vi "Subsistem Pengenalan Pola.vi"() -> ()   [LabVIEW 2011]
uses:
  <vilib>/vision/NI_Vision_Development_Module.lvlib
panel:
  in  "stop":bool
  in  "Color Plane":i32(ring)=1 items=["Red", "Green", "Blue", "Hue", "Saturation", "Luminance", "Value", "Intensity"]
  out "Objects":T1(array[cluster]) {"Aspect Ratio" format="%.2f"; "Orientation" format="%.2f"; "Area" format="%.2f"; "Object Center"."Y" format="%.2f"; "Object Center"."X" format="%.2f"}
  in  "Replace Value":sgl=255.0 format="%.2f"
  in  "Range":cluster{"Lower value":sgl, "Upper value":sgl}={"Lower value"=128.0, "Upper value"=255.0} {"Upper value" format="%.2f"; "Lower value" format="%.2f"}
  out "error vision 2":errorcluster
  in  "BERKAS / KAMERA":bool
  in  "Alamat Berkas":path=path "E:/D4 - TUGAS AKHIR/Programs/Praktikum/polman.png"
  out "Number of Objects":i32
  in  "Settings":T2={"Objects"=1, "Threshold"=128, "Reject Border"=FALSE, "Fill Holes"=FALSE, "Min Object Size"=FALSE, "Min Size"=100, "Max Object Size"=FALSE, "Max Size"=10000, "Show Search Area"=FALSE, "Show Center"=TRUE, "Show Bounding Box"=TRUE} {"Objects" items=["Bright Objects", "Dark Objects"]; "Threshold" min=1 max=999999999 step=1; "Max Size" min=1 max=999999999 step=1; "Min Size" min=1 max=999999999 step=1}
  out "Hasil \nKlasifikasi":T3(plugin-control)
  out "Hasil\nSegmentasi":T3(plugin-control)
  out "Citra \nHitam/Putih":T3(plugin-control)
  out "Citra Asli":T3(plugin-control)
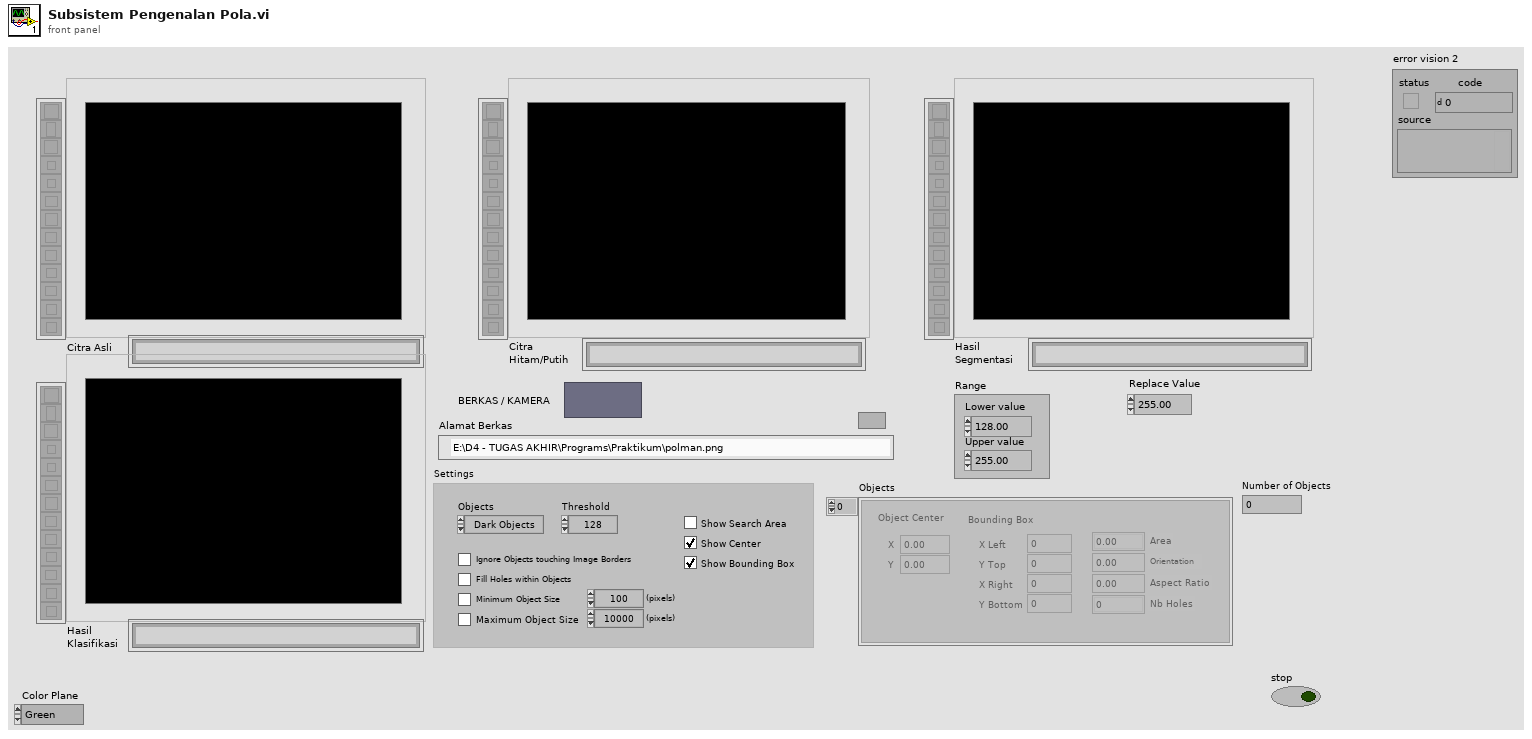
[diagram p1: front panel]
types:
  T1 = cluster{"Object Center":cluster{"X":sgl, "Y":sgl}, "Bounding Box":cluster{"X Left":i32, "Y Top":i32, "X Right":i32, "Y Bottom":i32}, "Area":sgl, "Orientation":sgl, "Aspect Ratio":sgl, "Nb Holes":i32}[]
  T2 = cluster{"Objects":u16, "Threshold":i32, "Reject Border":bool, "Fill Holes":bool, "Min Object Size":bool, "Min Size":i32, "Max Object Size":bool, "Max Size":i32, "Show Search Area":bool, "Show Center":bool, "Show Bounding Box":bool}
  T3 = typedef "IMAQ Image.ctl" = refnum<image>
  T4 = typedef "Image Type" = u32
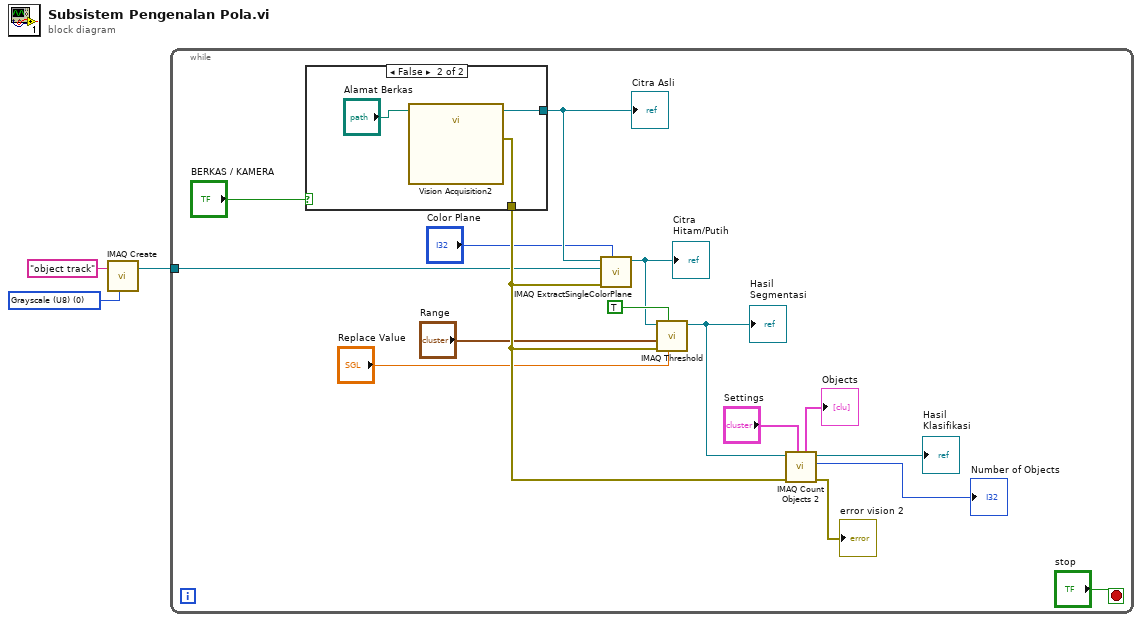
[diagram p0: block diagram]
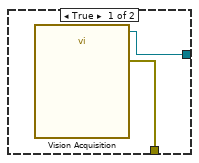
[diagram p2: hidden frame]
diagram:
  w2 = T4 0 items=["Grayscale (U8)", "Grayscale (I16)", "Grayscale (SGL)", "Complex (CSG)", "RGB (U32)", "HSL (U32)", "RGB (U64)", "Grayscale (U16)"] ("Image Type")
  n1 = call "IMAQ Create"("Image Name"="object track", "Image Type"=w2) -> ("New Image"=w1:T3)  [unwired: 3 in, 1 out]
  n2 = while {
    tunnel: w1 -> [w4]
    stop <- "stop" stop-if-true
    n3 = case shown="False" "BERKAS / KAMERA" {
      tunnel: [w20 w23] -> w19
      tunnel: [w21 w22] -> w13
      frame True {
        n4 = call "Vision Acquisition"() -> ("Image Out"=w20:T3, "error out"=w21:errorcluster)  [unwired: 25 in, 1 out]
      }
      frame False {
        n5 = call "Vision Acquisition2"("Image Path"="Alamat Berkas") -> ("Image Out"=w23:T3, "error out"=w22:errorcluster)  [unwired: 24 in, 1 out]
      }
    }
    "Citra Asli" <- w19
    n6 = call "IMAQ ExtractSingleColorPlane"("Color Plane"="Color Plane", "error in (no error)"=w13, "Image Dst"=w4, "Image Src"=w19) -> ("Image Dst Out"=w7:T3)  [unwired: 6 in, 1 out]
    "Citra \nHitam/Putih" <- w7
    n7 = call "IMAQ Threshold"("Replace Value"="Replace Value", "Keep/Replace Value (Replace)"=TRUE, "error in (no error)"=w13, "Range"="Range", "Image Src"=w7) -> ("Image Dst Out"=w6:T3)  [unwired: 5 in, 1 out]
    "Hasil\nSegmentasi" <- w6
    n8 = call "IMAQ Count Objects 2"("Settings"="Settings", "error in (no error)"=w13, "Image"=w6) -> ("error out"=→"error vision 2":errorcluster, "Number of Objects"=→"Number of Objects":i32, "Image Out"=→"Hasil \nKlasifikasi":T3, "Objects"=→"Objects":T1)  [unwired: 4 in, 1 out]
  }
